vi "SetControlValue.vi"(0 "vi":string, 1 "application reference (local)":refnum<vi>, 2 "vi ref":refnum<vi>, 3 "Signaling":bool=TRUE, 5 "ctrl":string, 7 "Value (JSON)":string, 9 "Value":variant, 11 "error in (no error)":errorcluster, 12 "control ref":refnum<vi>) -> (15 "error out":errorcluster)   [LabVIEW 2019, in "SetGetControlValue.lvlib"]
uses:
  SetGetControlValue.lvlib
  <vilib>/Utility/Data Type/NI_Data Type.lvlib
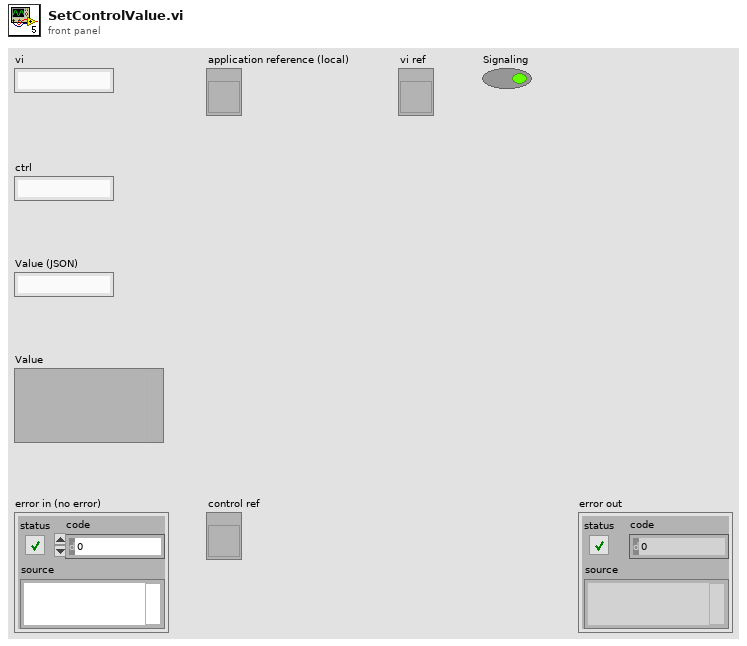
[diagram p1: front panel]
types:
  T1 = cluster{"ControlIndex":i32, "Control":refnum<vi>, "ArrayIndices":i32[]}[]
  T2 = typedef "NI_Data Type.lvlib/Data Type.ctl" = enum8{"Invalid Type", "Void", "I8", "I16", "I32", "I64", "U8", "U16", "U32", "U64", "Single Float", "Double Float", "Extended Float", "Single Complex", "Double Complex", "Extended Complex", "Enum U8", "Enum U16", "Enum U32", "Enum U64", "Single Float With Unit", "Double Float With Unit", "Extended Float With Unit", "Single Complex with Unit", "Double Complex with Unit", "Extended Complex with Unit", "Boolean", "String", "Path", "Picture", "Tag", "Array", "Cluster", "Variant", "LV Variant", "Waveform", "Timestamp", "Digital Waveform", "Digital Data", "ExpressData", "Refnum", "External Data", "VI", "Poly VI", "LabVIEW Class Instance", "Fixed Point", "Set Collection", "Map Collection"}
  T3 = cluster{"Type":enum16{"null", "number", "boolean", "string", "array", "object", ""}, "Value":variant}
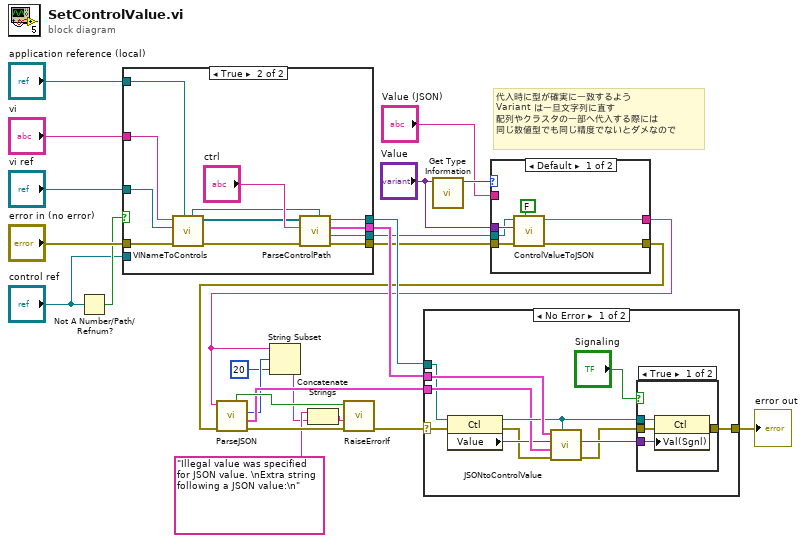
[diagram p0: block diagram]
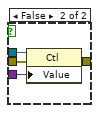
[diagram p3: hidden frame]
diagram:
  # "代入時に型が確実に一致するよう \nVariant は一旦文字列に直す\n配列やクラスタの一部へ代入する際には\n同じ数値型でも同じ精度でないとダメなので"
  n1 = Not A Number/Path/Refnum?(number/path/refnum="control ref") -> (NaN/Path/Refnum?=w2:bool)
  n2 = case shown="True" w2 {
    tunnel: "error in (no error)" -> [w26 w38]
    tunnel: "application reference (local)" -> [_ w37]
    tunnel: "vi" -> [_ w36]
    tunnel: [_ w32] -> w21
    tunnel: [w27 w31] -> w15
    tunnel: [w26 w30] -> w14
    tunnel: [w27 w29] -> w10
    tunnel: "vi ref" -> [_ w28]
    tunnel: "control ref" -> [w27 _]
    frame False {
    }
    frame True {
      n3 = call "VINameToControls.vi"("application reference (local)"=w37, "error in (no error)"=w38, "vi ref"=w28, "vi"=w36) -> ("error out"=w34:errorcluster, "FlattenControls[]"=w35:refnum<vi>[], "VI out"=w33:refnum<vi>)  [unwired: 5 in]
      n4 = call "ParseControlPath.vi"("VI"=w33, "error in (no error)"=w34, "control path string"="ctrl", "Controls[]"=w35) -> ("error out"=w30:errorcluster, "value element"=w29:refnum<vi>, "subcontrol path"=w32:T1, "control"=w31:refnum<vi>)  [unwired: 4 in]
    }
  }
  n5 = call <vilib>:"Get Type Information.vi"("variant"="Value") -> ("type"=w17:T2)  [unwired: 6 in, 4 out]
  n6 = case shown="Default" w17 {
    tunnel: [w43 w47] -> w6
    tunnel: "Value" -> [w44 _]
    tunnel: "Value (JSON)" -> [_ w47]
    tunnel: w14 -> [w42 w46]
    tunnel: [w41 w46] -> w13
    tunnel: w10 -> [w40 _]
    frame Default {
      n7 = call "ControlValueToJSON.vi"("UseEnum"=FALSE, "error in (no error)"=w42, "Value"=w44, "Control in"=w40) -> ("error out"=w41:errorcluster, "String"=w43:string)  [unwired: 6 in]
    }
    frame "Void" {
    }
  }
  n8 = call "ParseJSON.vi"("error in"=w13, "JSON string"=w6) -> ("error out"=w20:errorcluster, "Value"=w18:T3, "offset out"=w8:i32, "Remaining"=w19:bool)  [unwired: 5 in, 1 out]
  n9 = String Subset(string=w6, offset (0)=w8, length (rest)=20 ("length (rest)")) -> (substring=w3:string)
  n10 = Concatenate Strings("Illegal value was specified for JSON value. \nExtra string following a JSON value:\n" ("error source (\" \")"), w3) -> (w5:string)
  n11 = call "RaiseErrorIf.vi"("error in (no error)"=w20, "error message"=w5, "error? (true)"=w19) -> ("error out"=w12:errorcluster)  [unwired: 8 in]
  n12 = case shown="No Error" w12 {
    selector: w12 -> [w48 w67]
    tunnel: [w58 w67] -> w22
    tunnel: w21 -> [w57 _]
    tunnel: w18 -> [w52 _]
    tunnel: w15 -> [w49 _]
    frame No Error {
      n13 = property class="Ctl"(reference=w49, error in=w48) -> (reference out=w54:refnum<vi>, error out=w50:errorcluster, "Value"=w51:variant)
      n14 = call "JSONtoControlValue.vi"("control (for last item)"=w54, "error in"=w50, "Value"=w52, "Value in"=w51, "control path"=w57) -> ("error out"=w55:errorcluster, "Value out"=w56:variant)  [unwired: 5 in]
      n15 = case shown="True" "Signaling" {
        tunnel: w54 -> [w62 w66]
        tunnel: w56 -> [w61 w65]
        tunnel: w55 -> [w60 w64]
        tunnel: [w59 w63] -> w58
        frame True {
          n16 = property class="Ctl"(reference=w62, error in=w60, "Val(Sgnl)"=w61) -> (error out=w59:errorcluster)  [unwired: 1 out]
        }
        frame False {
          n17 = property class="Ctl"(reference=w66, error in=w64, "Value"=w65) -> (error out=w63:errorcluster)  [unwired: 1 out]
        }
      }
    }
    frame Error {
    }
  }
  "error out" <- w22
